vi "Card Number.vi"(2 "Random Number":dbl) -> (0 "Output":T1(array[cluster]))   [LabVIEW 2014]
uses:
  Card Used array.vi
panel:
  out "appended array":dbl[](array[numeric])
  out "size(s)":i32[](array[numeric])
  out "Output Cluster":T1(array[cluster])
  out "Solution Combination with 5 cards  and suits":dbl[][](array[numeric])
  out "Suits Array":dbl[][](array[numeric])
  out "Solution Combination with 5 cards":dbl[][](array[numeric])
  out "Solution Combination":dbl[][](array[numeric])
  out "Array":dbl[][](array[numeric])
  out "所有組合":dbl[][](array[numeric])
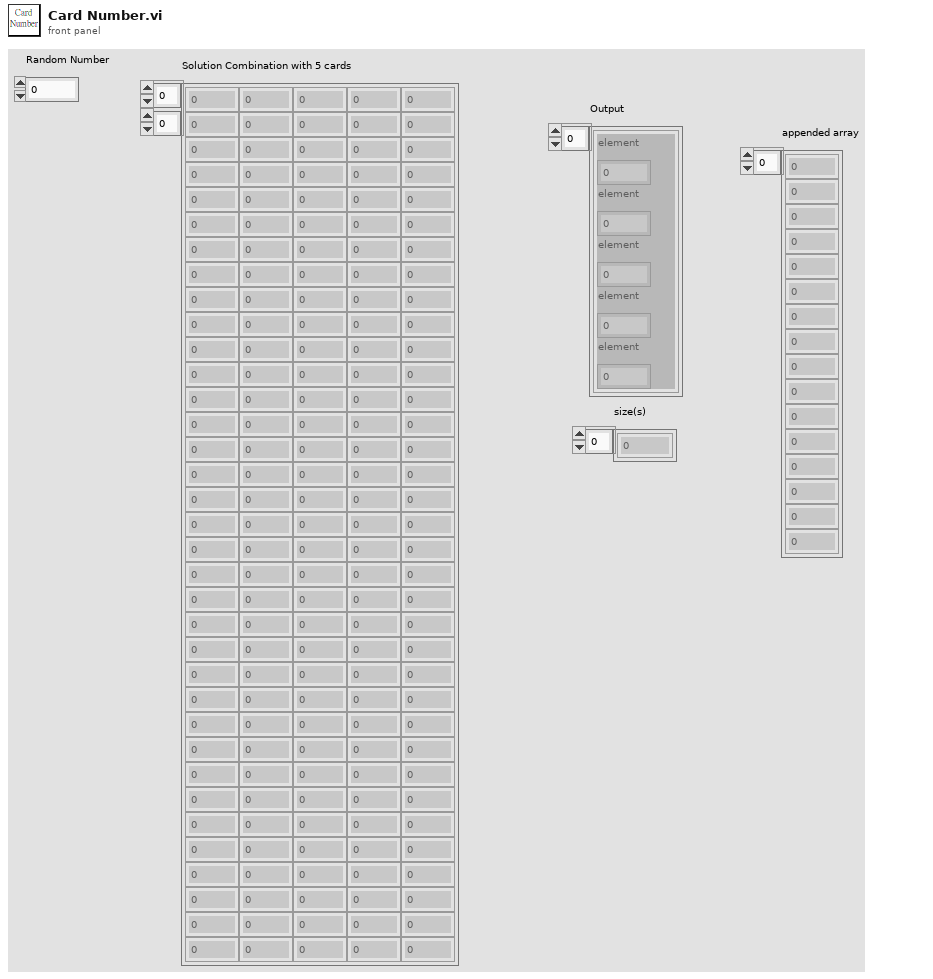
[diagram p1: front panel]
types:
  T1 = cluster{"element":dbl, "element":dbl, "element":dbl, "element":dbl, "element":dbl}[]
  T2 = cluster{"element":dbl, "element":dbl, "element":dbl, "element":dbl, "element":dbl}
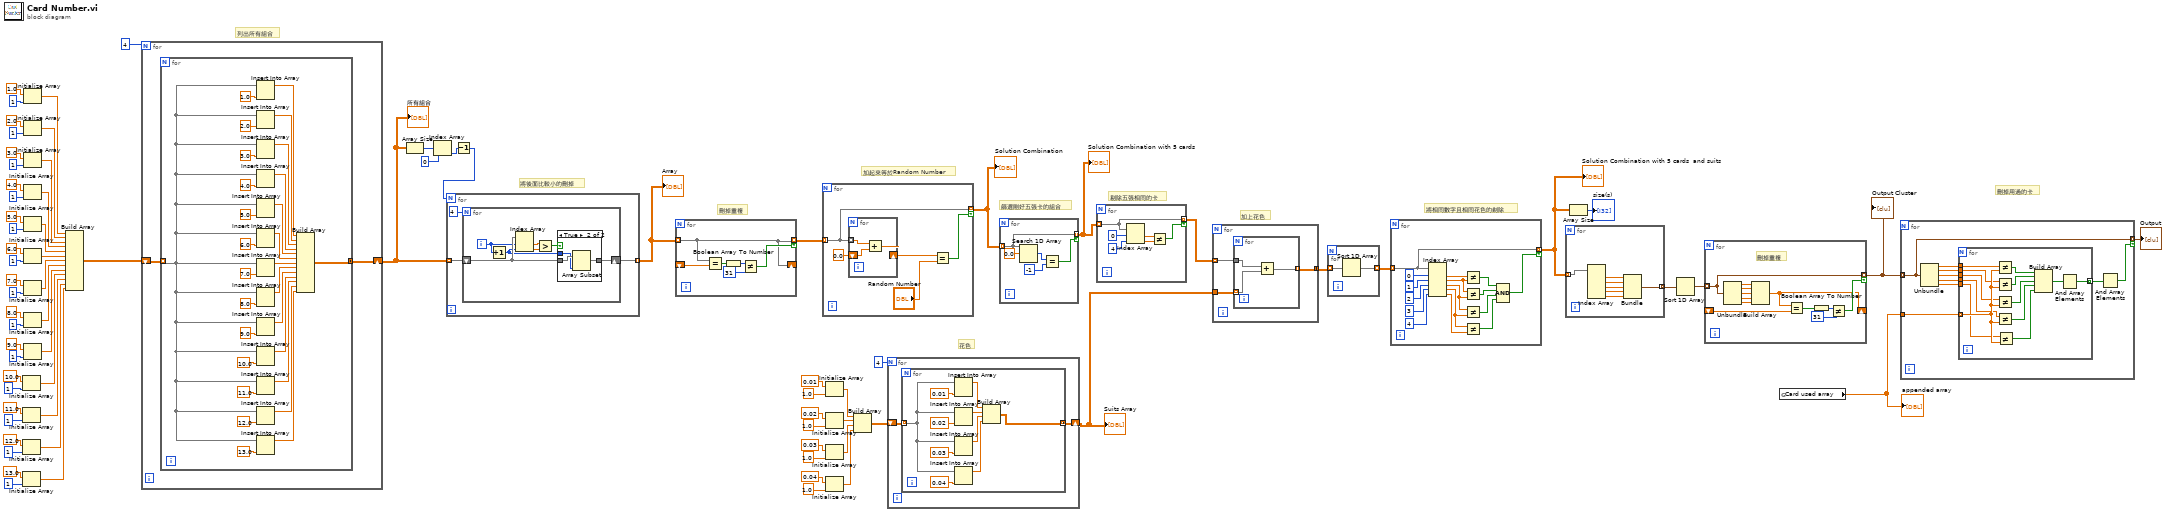
[diagram p0: block diagram]
diagram:
  # "刪掉用過的卡"
  # "將相同數字且相同花色的剃除"
  # "加上花色"
  # "花色"
  # "剔除五張相同的卡"
  # "列出所有組合"
  # "篩選剛好五張卡的組合"
  # "加起來等於Random Number"
  # "刪掉重複"
  # "將後面比較小的刪掉"
  n1 = Initialize Array(10.0 ("element"), 1 ("dimension size")) -> (w40:dbl[])
  n2 = Initialize Array(11.0 ("element"), 1 ("dimension size")) -> (w39:dbl[])
  n3 = Initialize Array(12.0 ("element"), 1 ("dimension size")) -> (w38:dbl[])
  n4 = Initialize Array(13.0 ("element"), 1 ("dimension size")) -> (w37:dbl[])
  n5 = Initialize Array(1.0 ("element"), 1 ("dimension size")) -> (w49:dbl[])
  n6 = Initialize Array(2.0 ("element"), 1 ("dimension size")) -> (w48:dbl[])
  n7 = Initialize Array(3.0 ("element"), 1 ("dimension size")) -> (w47:dbl[])
  n8 = Initialize Array(4.0 ("element"), 1 ("dimension size")) -> (w46:dbl[])
  n9 = Initialize Array(5.0 ("element"), 1 ("dimension size")) -> (w45:dbl[])
  n10 = Initialize Array(6.0 ("element"), 1 ("dimension size")) -> (w44:dbl[])
  n11 = Initialize Array(7.0 ("element"), 1 ("dimension size")) -> (w43:dbl[])
  n12 = Initialize Array(8.0 ("element"), 1 ("dimension size")) -> (w42:dbl[])
  n13 = Initialize Array(9.0 ("element"), 1 ("dimension size")) -> (w41:dbl[])
  n14 = Build Array(w49, w48, w47, w46, w45, w44, w43, w42, w41, w40, w39, w38, w37) -> (w36:dbl[][])
  n15 = for {
    N: 4 -> [_]
    shift-right: [w76] -> w31
    shift-left: w36 -> [w77]
    n16 = for {
      tunnel: w77 -> [w92] mode=indexing
      tunnel: [w78] -> w76 mode=concatenating
      n17 = Insert Into Array(array=w92, new element=10.0 ("new element/subarray")) -> (w82:dbl[])  [unwired: 1 in]
      n18 = Insert Into Array(array=w92, new element=11.0 ("new element/subarray")) -> (w81:dbl[])  [unwired: 1 in]
      n19 = Insert Into Array(array=w92, new element=12.0 ("new element/subarray")) -> (w80:dbl[])  [unwired: 1 in]
      n20 = Insert Into Array(array=w92, new element=13.0 ("new element/subarray")) -> (w79:dbl[])  [unwired: 1 in]
      n21 = Insert Into Array(array=w92, new element=1.0 ("new element/subarray")) -> (w91:dbl[])  [unwired: 1 in]
      n22 = Insert Into Array(array=w92, new element=2.0 ("new element/subarray")) -> (w90:dbl[])  [unwired: 1 in]
      n23 = Insert Into Array(array=w92, new element=3.0 ("new element/subarray")) -> (w89:dbl[])  [unwired: 1 in]
      n24 = Insert Into Array(array=w92, new element=4.0 ("new element/subarray")) -> (w88:dbl[])  [unwired: 1 in]
      n25 = Insert Into Array(array=w92, new element=5.0 ("new element/subarray")) -> (w87:dbl[])  [unwired: 1 in]
      n26 = Insert Into Array(array=w92, new element=6.0 ("new element/subarray")) -> (w86:dbl[])  [unwired: 1 in]
      n27 = Insert Into Array(array=w92, new element=7.0 ("new element/subarray")) -> (w85:dbl[])  [unwired: 1 in]
      n28 = Insert Into Array(array=w92, new element=8.0 ("new element/subarray")) -> (w84:dbl[])  [unwired: 1 in]
      n29 = Insert Into Array(array=w92, new element=9.0 ("new element/subarray")) -> (w83:dbl[])  [unwired: 1 in]
      n30 = Build Array(w91, w90, w89, w88, w87, w86, w85, w84, w83, w82, w81, w80, w79) -> (w78:dbl[][])
    }
  }
  "所有組合" <- w31
  n31 = Array Size(array=w31) -> (size(s)=w34:i32[])
  n32 = Index Array(array=w34, index=0) -> (element=w32:i32)
  n33 = Decrement(x=w32) -> (x-1=w30:i32)
  n34 = for {
    N: w30 -> [_]
    tunnel: w31 -> [w108] mode=indexing
    tunnel: [w107] -> w29 mode=indexing
    n35 = for {
      N: 4 -> [_]
      shift-right: [w111] -> w107
      shift-left: w108 -> [w112]
      i -> [w110]
      n36 = Increment(x=w110) -> (x+1=w109:i32)
      n37 = Index Array(array=w112, index #1=w110, index #2=w109) -> (element #1=w115:dbl, element #2=w114:dbl)
      n38 = Greater?(x=w115, y=w114) -> (0:w113:bool)
      n39 = case shown="True" w113 {
        tunnel: w112 -> [w116 w119]
        tunnel: [w116 w118] -> w111
        tunnel: w109 -> [_ w117]
        frame False {
        }
        frame True {
          n40 = Array Subset(array=w119, length=w117) -> (w118:dbl[])  [unwired: 1 in]
        }
      }
    }
  }
  "Array" <- w29
  n41 = for {
    tunnel: w29 -> [w121] mode=indexing
    shift-right: [w121] -> _
    shift-left: _ -> [w120]
    tunnel: [w121] -> w28 mode=indexing if=w122
    n42 = Equal?(x=w121, y=w120) -> (x = y?=w125:bool[])
    n43 = Boolean Array To Number(Boolean array=w125) -> (number=w124:u32)
    n44 = Not Equal?(x=w124, y=u32 31) -> (x != y?=w122:bool)
  }
  n45 = for {
    tunnel: w28 -> [w128] mode=indexing
    tunnel: [w128] -> w27 mode=indexing if=w127
    n46 = for {
      tunnel: w128 -> [w133] mode=indexing
      shift-right: [w132] -> w129
      shift-left: 0.0 -> [w131]
      n47 = Add(x=w133, y=w131) -> (x+y=w132:dbl)
    }
    n48 = Equal?(x=w129, y="Random Number") -> (x = y?=w127:bool)
  }
  "Solution Combination" <- w27
  n49 = Initialize Array(0.01 ("element"), 1.0 ("dimension size")) -> (w18:dbl[])
  n50 = Initialize Array(0.02 ("element"), 1.0 ("dimension size")) -> (w17:dbl[])
  n51 = Initialize Array(0.03 ("element"), 1.0 ("dimension size")) -> (w16:dbl[])
  n52 = Initialize Array(0.04 ("element"), 1.0 ("dimension size")) -> (w15:dbl[])
  n53 = Build Array(w18, w17, w16, w15) -> (w13:dbl[][])
  n54 = for {
    N: 4 -> [_]
    shift-right: [w134] -> w12
    shift-left: w13 -> [w135]
    n55 = for {
      tunnel: w135 -> [w137] mode=indexing
      tunnel: [w136] -> w134 mode=concatenating
      n56 = Insert Into Array(array=w137, new element=0.01 ("new element/subarray")) -> (w141:dbl[])  [unwired: 1 in]
      n57 = Insert Into Array(array=w137, new element=0.02 ("new element/subarray")) -> (w140:dbl[])  [unwired: 1 in]
      n58 = Insert Into Array(array=w137, new element=0.03 ("new element/subarray")) -> (w139:dbl[])  [unwired: 1 in]
      n59 = Insert Into Array(array=w137, new element=0.04 ("new element/subarray")) -> (w138:dbl[])  [unwired: 1 in]
      n60 = Build Array(w141, w140, w139, w138) -> (w136:dbl[][])
    }
  }
  "Suits Array" <- w12
  n61 = for {
    tunnel: w27 -> [w147] mode=indexing
    tunnel: [w147] -> w11 mode=indexing if=w146
    n62 = Search 1D Array(1D array=w147, element=0.0) -> (index of element=w149:i32)  [unwired: 1 in]
    n63 = Equal?(x=w149, y=-1) -> (x = y?=w146:bool)
  }
  "Solution Combination with 5 cards" <- w11
  n64 = for {
    tunnel: [w151] -> w10 mode=indexing if=w154
    tunnel: w11 -> [w151] mode=indexing
    n65 = Index Array(array=w151, index #1=0 ("index"), index #2=4 ("index")) -> (element #1=w153:dbl, element #2=w152:dbl)
    n66 = Not Equal?(x=w153, y=w152) -> (x != y?=w154:bool)
  }
  n67 = for {
    tunnel: w10 -> [w158] mode=indexing
    tunnel: w12 -> [w159]
    tunnel: [w157] -> w5 mode=concatenating
    n68 = for {
      tunnel: w159 -> [w161] mode=indexing
      tunnel: w158 -> [w162]
      tunnel: [w160] -> w157 mode=indexing
      n69 = Add(x=w162, y=w161) -> (x+y=w160:dbl[])
    }
  }
  n70 = for {
    tunnel: [w164] -> w9 mode=indexing
    tunnel: w5 -> [w163] mode=indexing
    n71 = Sort 1D Array(array=w163) -> (sorted array=w164:dbl[])
  }
  n72 = for {
    tunnel: w9 -> [w167] mode=indexing
    tunnel: [w167] -> w4 mode=indexing if=w166
    n73 = Index Array(array=w167, index #1=0 ("index"), index #2=1 ("index"), index #3=2 ("index"), index #4=3 ("index"), index #5=4 ("index")) -> (element #1=w176:dbl, element #2=w175:dbl, element #3=w174:dbl, element #4=w173:dbl, element #5=w172:dbl)
    n74 = Not Equal?(x=w176, y=w175) -> (x != y?=w171:bool)
    n75 = Not Equal?(x=w175, y=w174) -> (x != y?=w170:bool)
    n76 = Not Equal?(x=w174, y=w173) -> (x != y?=w169:bool)
    n77 = Not Equal?(x=w173, y=w172) -> (x != y?=w168:bool)
    n78 = Compound Arithmetic op=AND(w171, w170, w169, w168) -> (w166:bool)
  }
  "Solution Combination with 5 cards  and suits" <- w4
  n79 = for {
    tunnel: [w182] -> w7 mode=indexing
    tunnel: w4 -> [w181] mode=indexing
    n80 = Index Array(array=w181) -> (element #1=w187:dbl, element #2=w186:dbl, element #3=w185:dbl, element #4=w184:dbl, element #5=w183:dbl)  [unwired: 5 in]
    n81 = Bundle("element"=w187, "element"=w186, "element"=w185, "element"=w184, "element"=w183) -> (w182:T2)  [unwired: 1 in]
  }
  n82 = Array Size(array=w4) -> (size(s)=→"size(s)":i32[])
  n83 = Sort 1D Array(array=w7) -> (sorted array=w6:T1)
  n84 = for {
    tunnel: w6 -> [w188] mode=indexing
    shift-right: [w189] -> _
    shift-left: _ -> [w199]
    tunnel: [w188] -> w3 mode=indexing if=w195
    # "刪掉重複"
    n85 = Unbundle(w188) -> ("element"=w194:dbl, "element"=w190:dbl, "element"=w191:dbl, "element"=w192:dbl, "element"=w193:dbl)
    n86 = Build Array(w194, w190, w191, w192, w193) -> (w189:dbl[])
    n87 = Equal?(x=w189, y=w199) -> (x = y?=w198:bool[])
    n88 = Boolean Array To Number(Boolean array=w198) -> (number=w197:u32)
    n89 = Not Equal?(x=w197, y=u32 31) -> (x != y?=w195:bool)
  }
  "Output Cluster" <- w3
  n90 = global read "Card Used array.vi" "Card used array"() -> (w1:dbl[])
  "appended array" <- w1
  n91 = for {
    tunnel: w3 -> [w202] mode=indexing
    tunnel: w1 -> [w208]
    tunnel: [w202] -> w2 mode=indexing if=w200
    n92 = Unbundle(w202) -> ("element"=w207:dbl, "element"=w206:dbl, "element"=w205:dbl, "element"=w204:dbl, "element"=w203:dbl)
    n93 = for {
      tunnel: w208 -> [w220] mode=indexing
      tunnel: w207 -> [w221]
      tunnel: w206 -> [w219]
      tunnel: w205 -> [w218]
      tunnel: w204 -> [w217]
      tunnel: w203 -> [w216]
      tunnel: [w209] -> w201 mode=indexing
      n94 = Not Equal?(x=w221, y=w220) -> (x != y?=w215:bool)
      n95 = Not Equal?(x=w219, y=w220) -> (x != y?=w214:bool)
      n96 = Not Equal?(x=w218, y=w220) -> (x != y?=w213:bool)
      n97 = Not Equal?(x=w217, y=w220) -> (x != y?=w212:bool)
      n98 = Not Equal?(x=w216, y=w220) -> (x != y?=w211:bool)
      n99 = Build Array(w215, w214, w213, w212, w211) -> (w210:bool[])
      n100 = And Array Elements(Boolean array=w210) -> (logical AND=w209:bool)
    }
    n101 = And Array Elements(Boolean array=w201) -> (logical AND=w200:bool)
  }
  "Output" <- w2
